vi "VISCOSITY_autoranging.vi"(1 "stabilization (ms)":u32=15000, 5 "TorqueOffset":dbl=-1.0, 6 "DataPoints":i32=10, 7 "GUID":string, 8 "Zero?":bool=TRUE, 9 "LogData?":bool=TRUE, 10 "rpm setpoint":i32=180) -> (0 "Torque% Offset":dbl, 2 "cP_mean":dbl format="%0.2f", 3 "TorqueArray":dbl[](array[numeric]), 4 "cP_Array":dbl[](array[numeric]))   [LabVIEW 2019]
uses:
  Brookfield_type-def.ctl
  <vilib>/Instr/_visa.llb/VISA Flush IO Buffer Mask.ctl
  <vilib>/Utility/error.llb/DialogType.ctl
  <vilib>/Analysis/baseanly.llb/Mean (DBL).vi
  <vilib>/Analysis/NI_AALBase.lvlib
panel:
  out "ReconnectAttempts":i32
  out "log_string":string
  out "error (enable read)":errorcluster
  out "TempArray":dbl[](array[numeric])
  out "error out":errorcluster
  out "Enum":T1
  out "temp":dbl
  out "torque%":dbl
  out "Control Circuitry Enabled":bool
  out "Motor On":bool
  out "Motor Stopped":bool
  out "Auto-zero Complete":bool
  out "Motor Circuit Error":bool
  out "Diagnostics Error":bool
  out "Invalid Command Received":bool
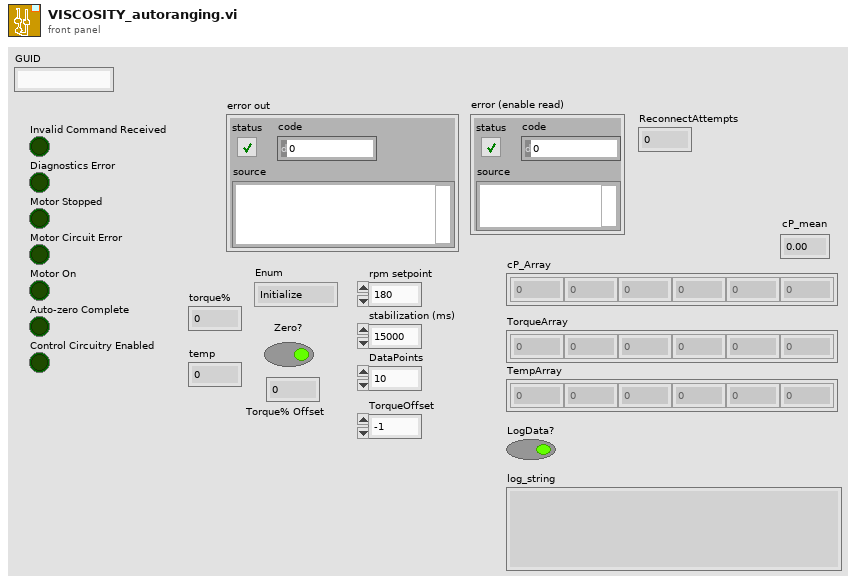
[diagram p1: front panel]
types:
  T1 = typedef "Brookfield_type-def.ctl" = enum16{"Initialize", "Enable", "Ready", "Zero", "Set Speed", "Read", "Stop Motor", "Error", "Disconnect"}
  T2 = enum16{"open", "replace", "create", "open or create", "replace or create", "replace or create with confirmation"}
  T3 = typedef "VISA Flush IO Buffer Mask.ctl" = u16
  T4 = typedef "DialogType.ctl" = u16
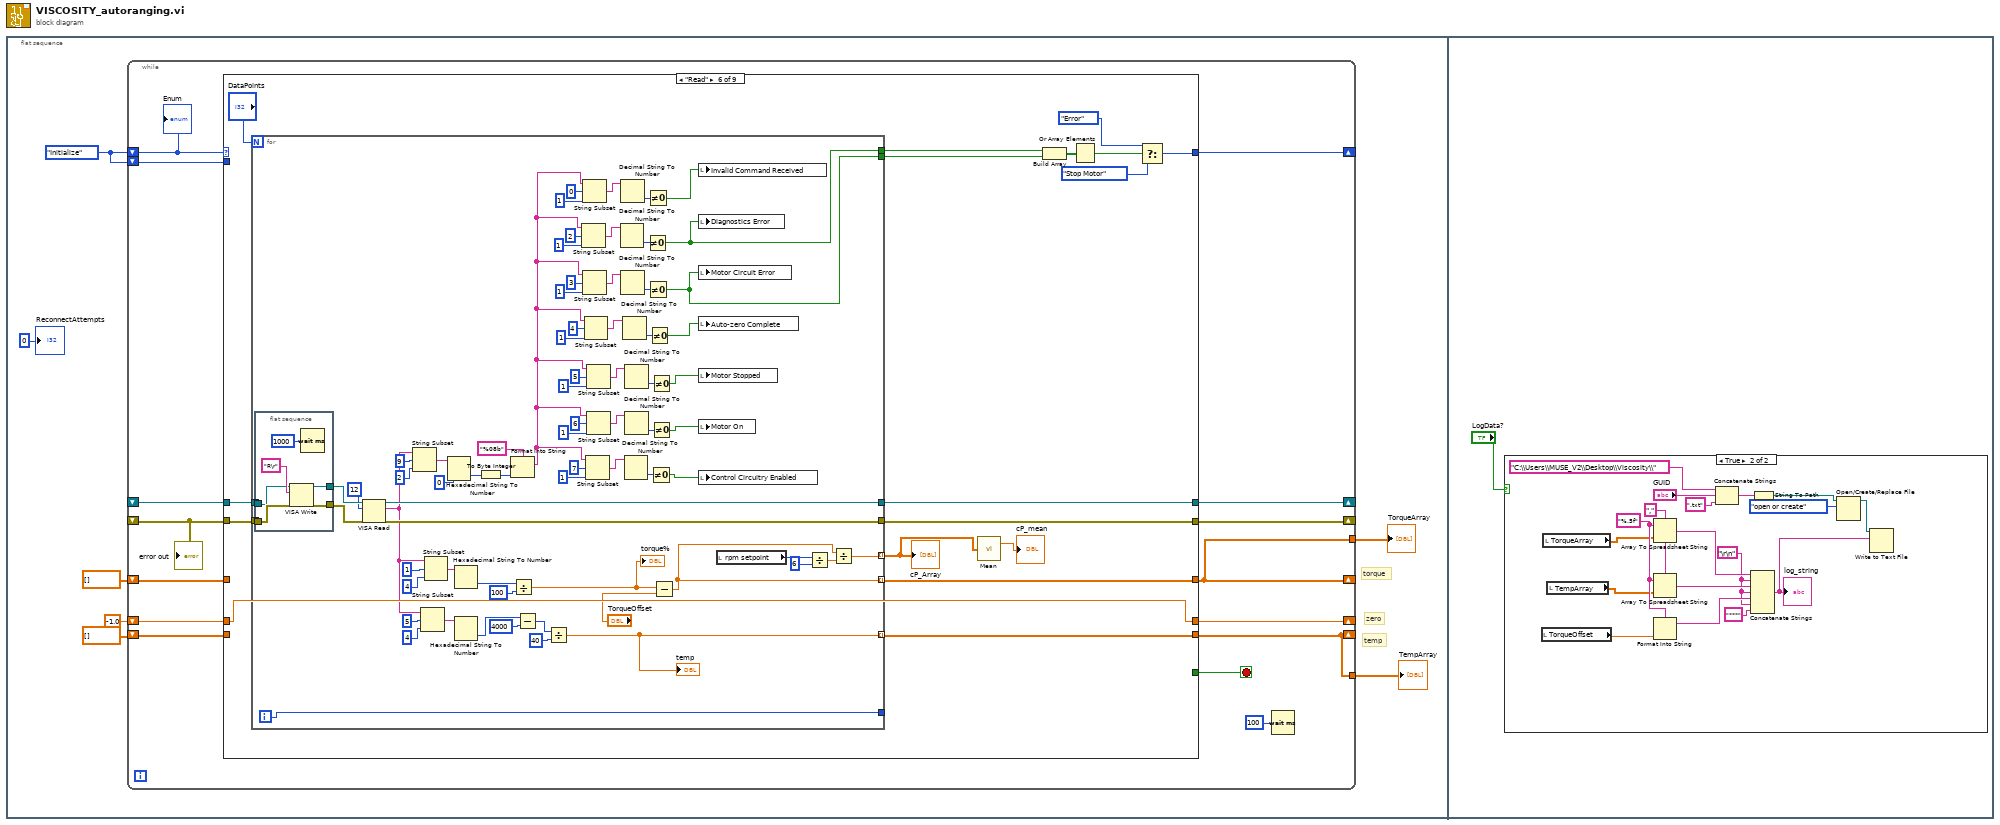
[diagram p0: block diagram]
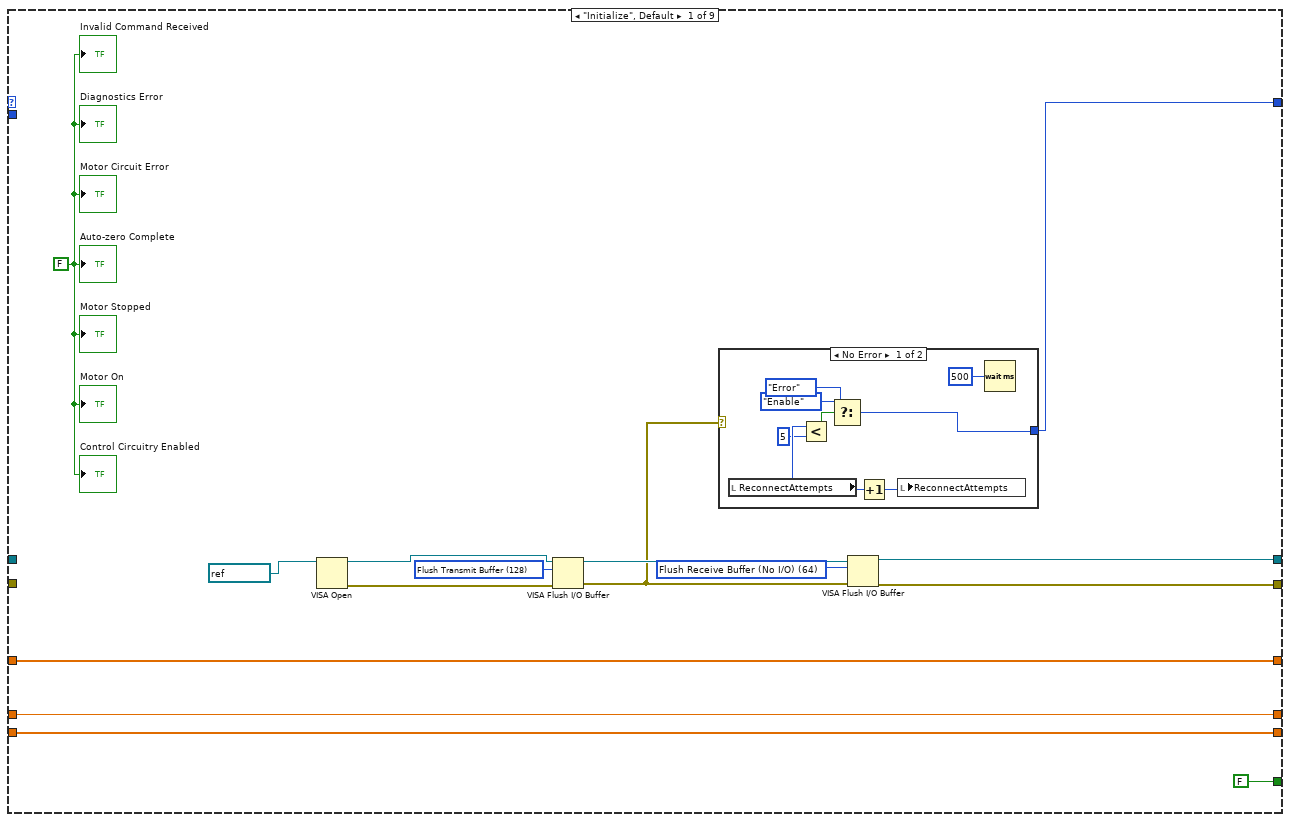
[diagram p2: hidden frame]
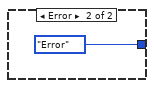
[diagram p3: hidden frame]
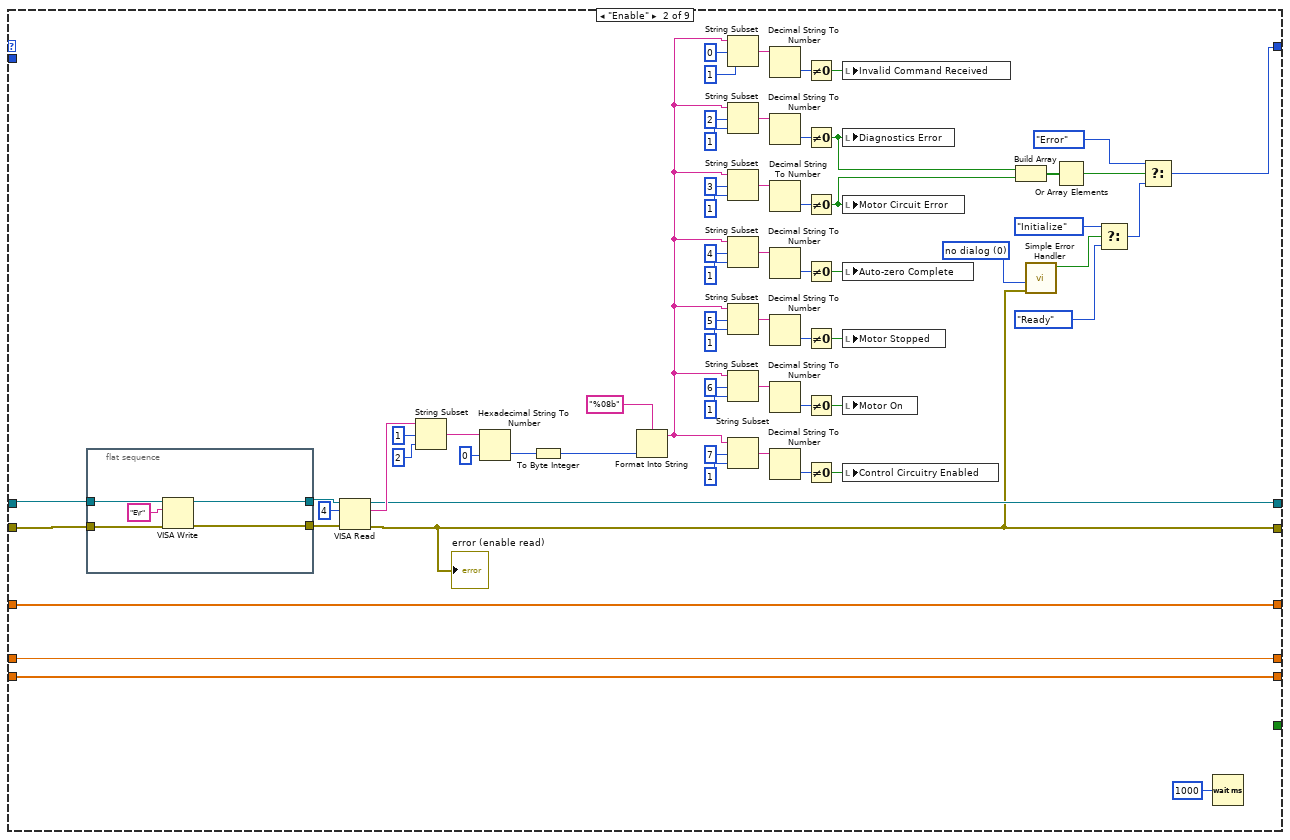
[diagram p4: hidden frame]
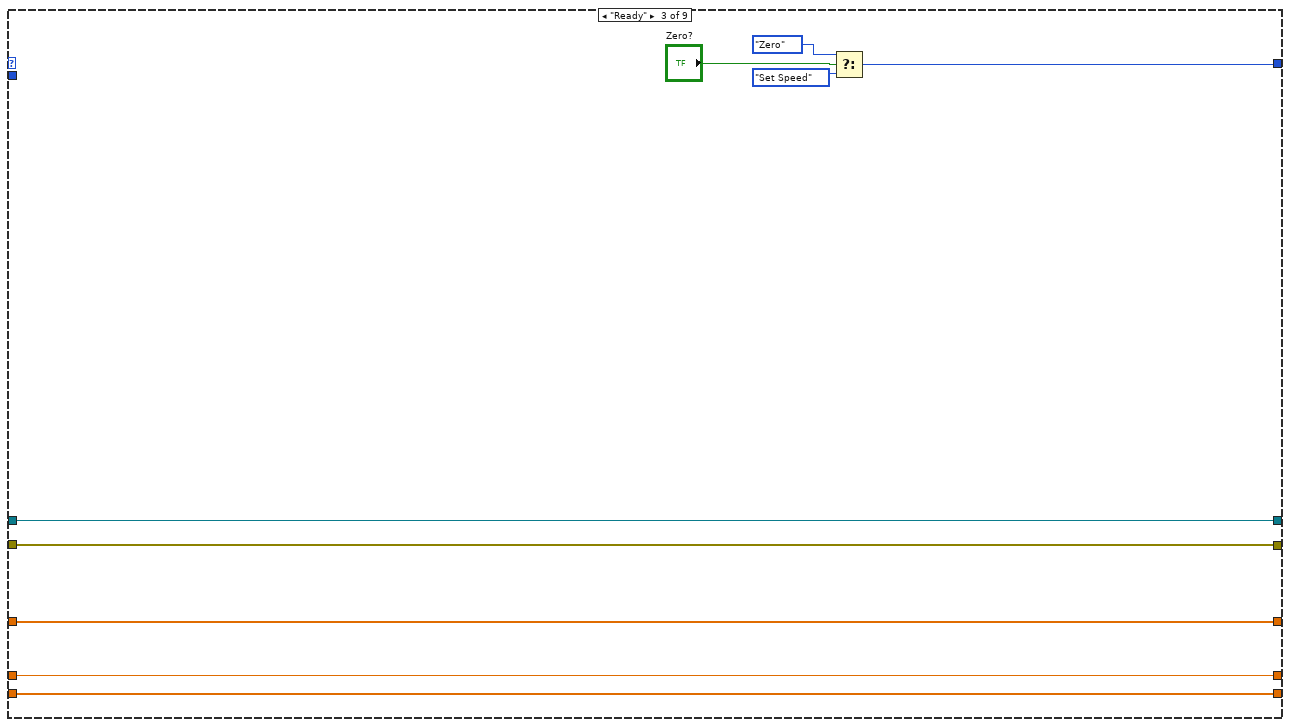
[diagram p5: hidden frame]
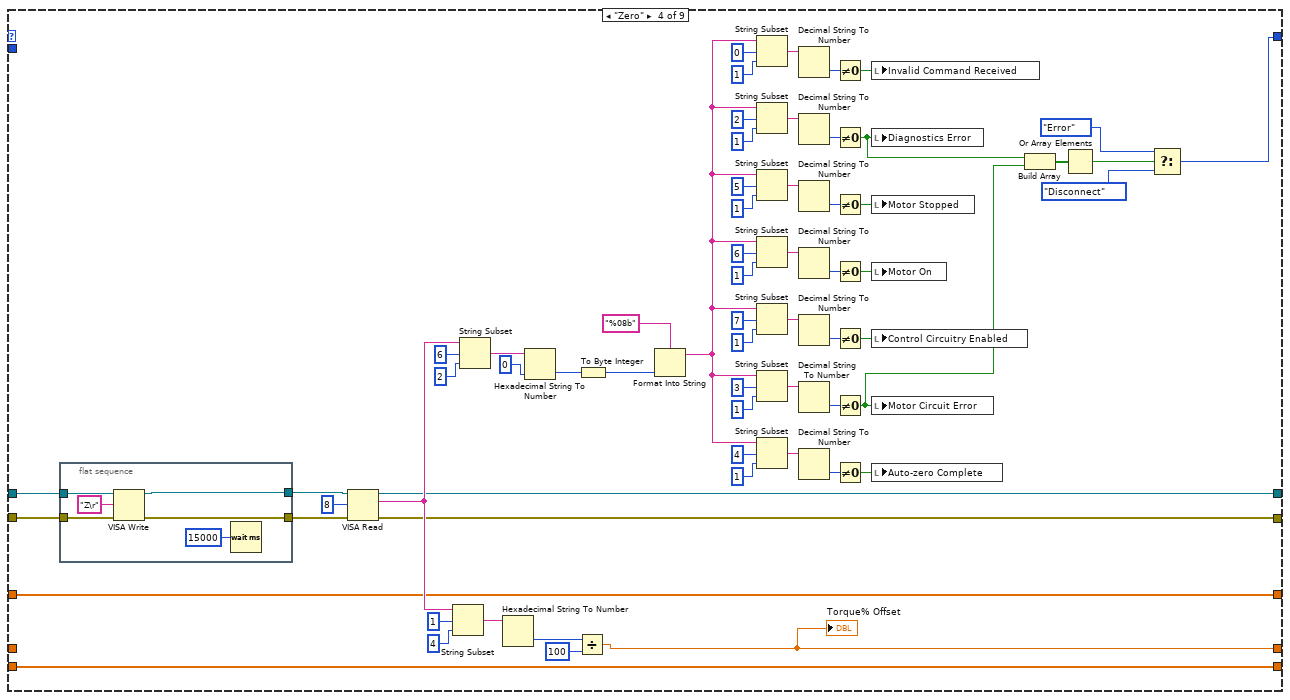
[diagram p6: hidden frame]
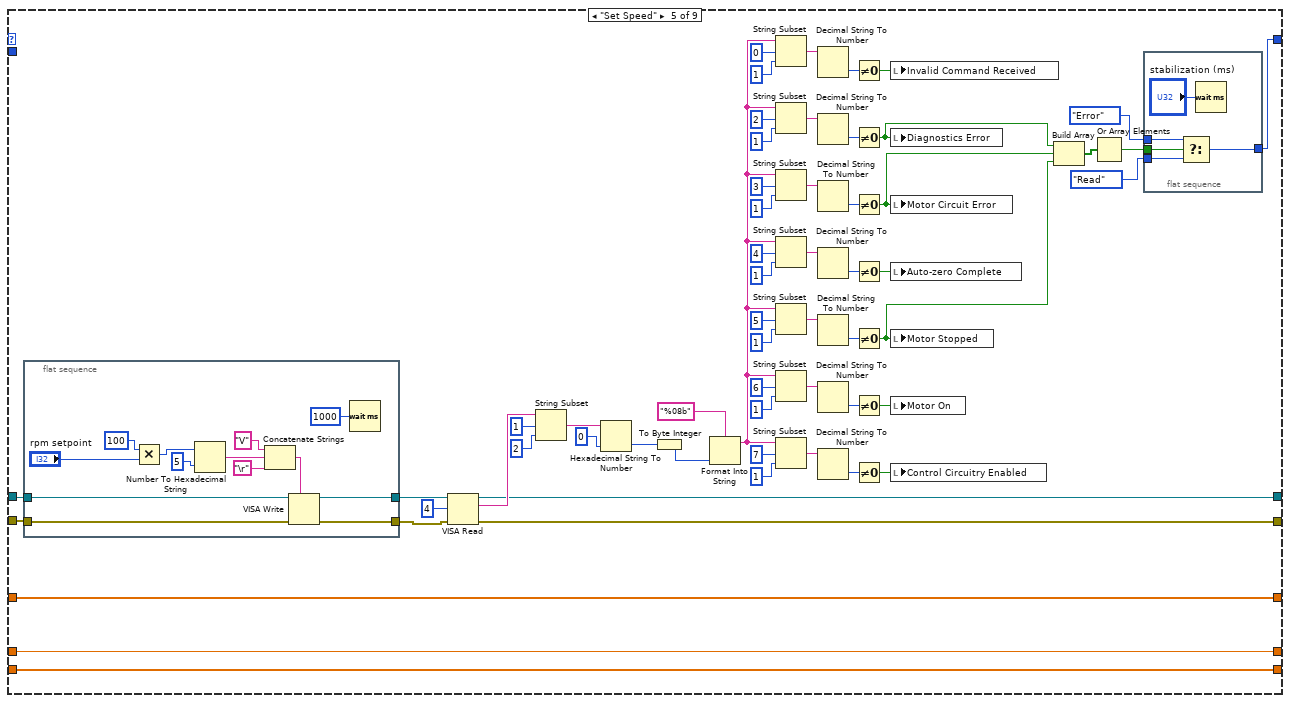
[diagram p7: hidden frame]
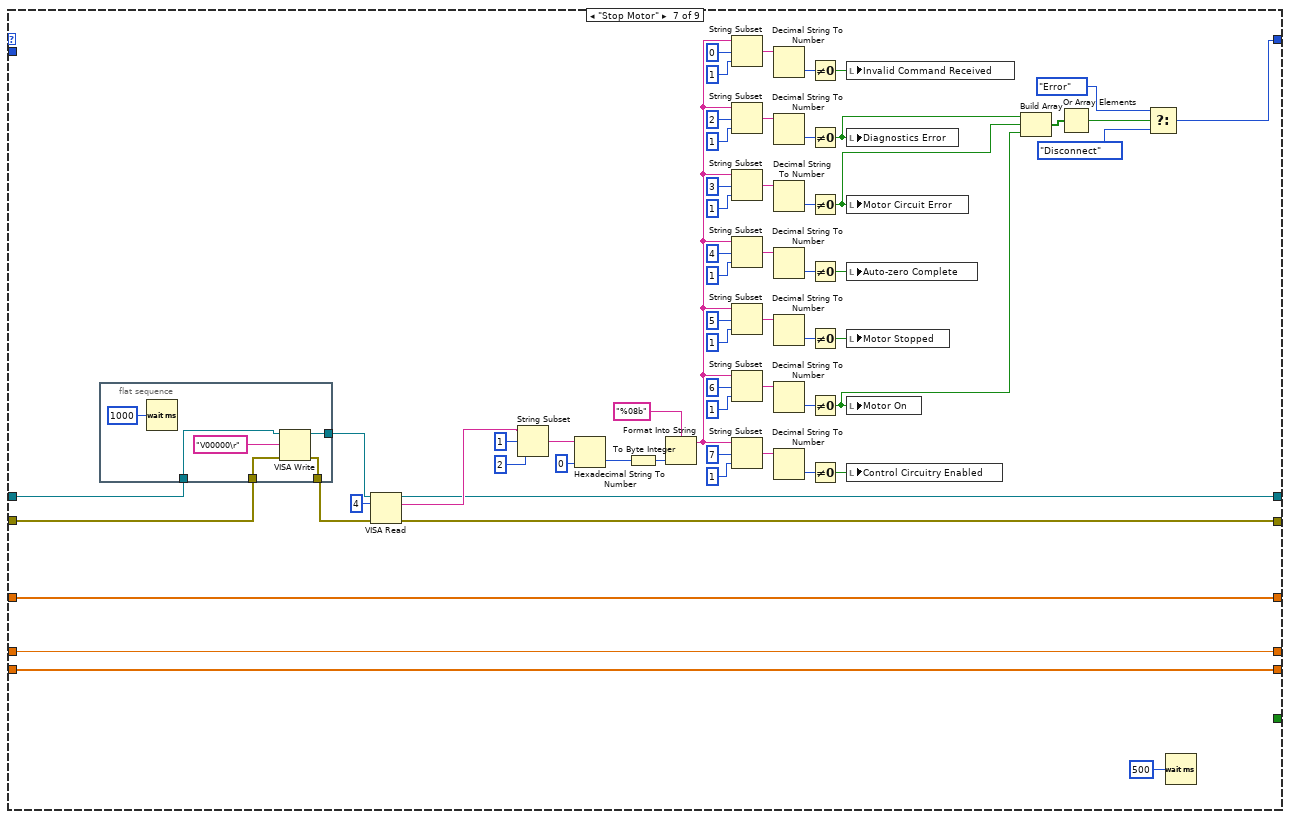
[diagram p8: hidden frame]
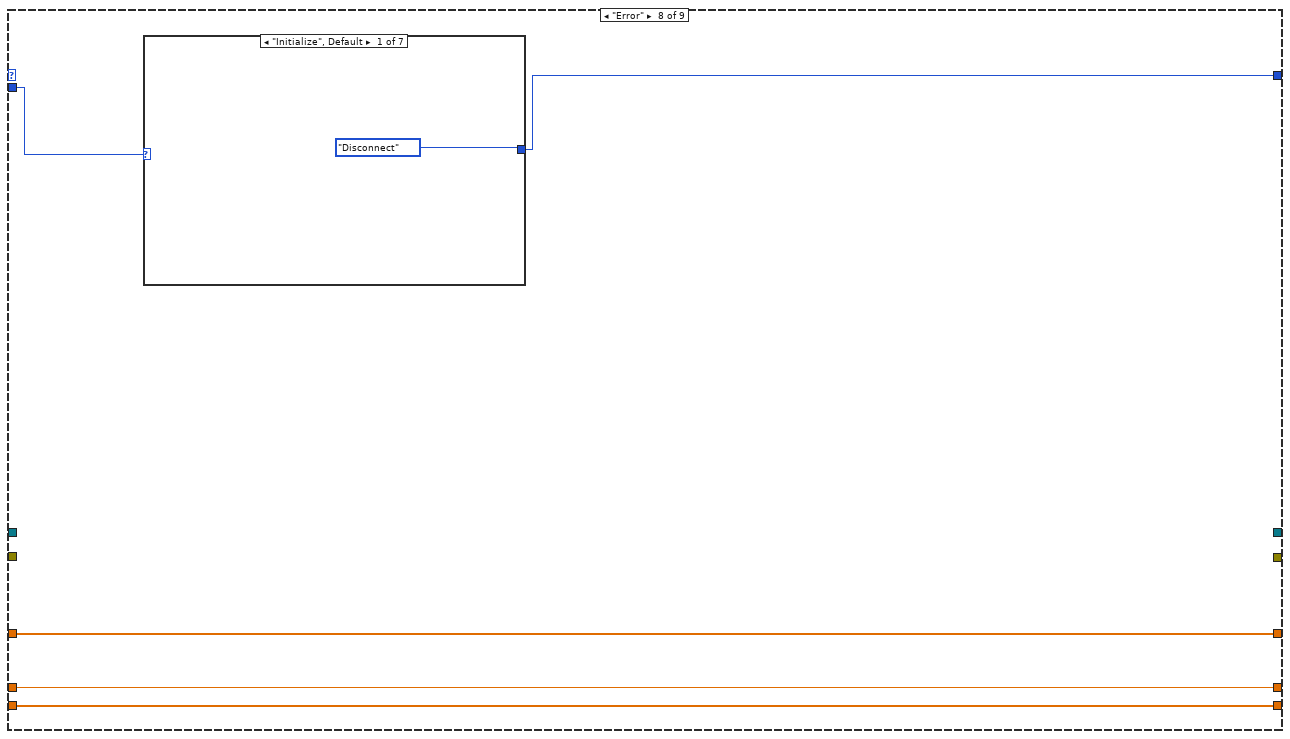
[diagram p9: hidden frame]
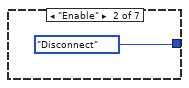
[diagram p10: hidden frame]
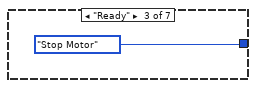
[diagram p11: hidden frame]
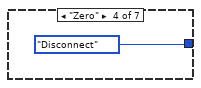
[diagram p12: hidden frame]
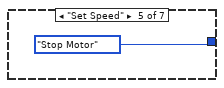
[diagram p13: hidden frame]
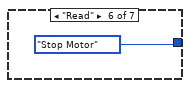
[diagram p14: hidden frame]
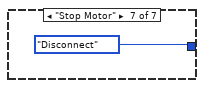
[diagram p15: hidden frame]
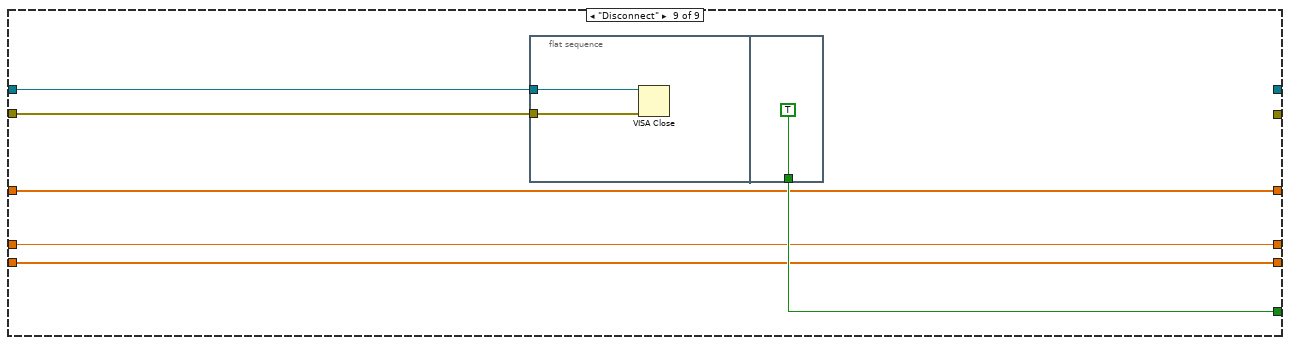
[diagram p16: hidden frame]
diagram:
  n1 = flat-sequence {
    frame #0 {
      w7 = Brookfield_type-def."Initialize"
      # "temp"
      # "zero"
      # "torque"
      n2 = while {
        shift-right: [w16] -> _
        shift-left: w7 -> [w22]
        shift-right: [w21] -> _
        shift-left: _ -> [w19]
        shift-right: [w20] -> _
        shift-left: _ -> [w18]
        shift-right: [w9] -> _
        shift-left: dbl[] [] -> [w14]
        shift-right: [w8] -> _
        shift-left: dbl[] [] -> [w11]
        shift-left: w7 -> [w15]
        shift-right: [w12] -> _
        shift-left: -1.0 -> [w13]
        tunnel: [w9] -> w3
        tunnel: [w8] -> w2
        stop <- w17 stop-if-true
        n3 = case shown="\"Read\"" w22 {
          tunnel: [w24 w65 w120 w135 w211 w288 w383 _ _] -> w21
          tunnel: [w23 w48 w121 w136 w212 w287 w384 _ _] -> w20
          tunnel: w19 -> [_ w110 w120 w138 w197 w276 w370 _ w450]
          tunnel: w18 -> [_ w109 w121 w137 w198 w277 w371 _ w449]
          tunnel: [FALSE _ _ _ _ _ _ _ w448] -> w17
          tunnel: [w34 w59 w117 w128 w206 w283 w378 w437 _] -> w16
          tunnel: [w33 w58 w124 w127 w201 w279 w374 w436 w447] -> w9
          tunnel: [w31 w56 w122 w126 w199 w280 w372 w434 w445] -> w8
          tunnel: [w32 w57 w123 w125 w200 w278 w373 w435 w446] -> w12
          tunnel: w15 -> [_ _ _ _ _ _ _ w433 _]
          tunnel: w14 -> [w33 w58 w124 w127 w201 _ w374 w436 w447]
          tunnel: w13 -> [w32 w57 w123 _ w200 w278 w373 w435 w446]
          tunnel: w11 -> [w31 w56 w122 w126 w199 _ w372 w434 w445]
          frame "Initialize", Default {
            w25 = T3 64 items=["Flush Receive Buffer"=16, "Write Transmit Buffer to Device"=32, "Flush Receive Buffer (No I/O)"=64, "Flush Transmit Buffer"=128] ("Mask")
            w28 = T3 128 items=["Flush Receive Buffer"=16, "Write Transmit Buffer to Device"=32, "Flush Receive Buffer (No I/O)"=64, "Flush Transmit Buffer"=128] ("Mask")
            w36 = FALSE
            n4 = VISA Open(VISA resource name=refnum<visa-resource-name> "COM5" ("Conductivity Port")) -> (VISA resource name=w29:refnum<visa-resource-name>, error out=w30:errorcluster)  [unwired: 4 in]
            n5 = VISA Flush I/O Buffer(VISA resource name=w29, mask (16)=w28, error in (no error)=w30) -> (VISA resource name out=w27:refnum<visa-resource-name>, error out=w26:errorcluster)
            n6 = case shown="No Error" w26 {
              tunnel: [w40 Brookfield_type-def."Error"] -> w34
              frame No Error {
                n7 = local read "ReconnectAttempts"() -> (w43:i32)
                n8 = Less?(x=w43, y=5) -> (x < y?=w41:bool)
                n9 = Select(t=Brookfield_type-def."Enable", s=w41, f=Brookfield_type-def."Error") -> (s? t:f=w40:T1)
                n10 = Increment(x=w43) -> (x+1=w44:i32)
                n11 = local write "ReconnectAttempts"(w44) -> ()
                n12 = Wait (ms)(milliseconds to wait=u32 500) -> ()  [unwired: 1 out]
              }
              frame Error {
              }
            }
            n13 = VISA Flush I/O Buffer(VISA resource name=w27, mask (16)=w25, error in (no error)=w26) -> (VISA resource name out=w24:refnum<visa-resource-name>, error out=w23:errorcluster)
            "Invalid Command Received" <- w36
            "Diagnostics Error" <- w36
            "Motor Circuit Error" <- w36
            "Auto-zero Complete" <- w36
            "Motor Stopped" <- w36
            "Motor On" <- w36
            "Control Circuitry Enabled" <- w36
          }
          frame "Enable" {
            w50 = T4 0 items=["no dialog", "OK message", "continue or stop message", "OK message + warnings", "continue/stop + warnings"] ("type of dialog (OK msg:1)")
            n14 = flat-sequence {
              tunnel: w110 -> [w114]
              tunnel: w109 -> [w113]
              tunnel: [w112] -> w49
              tunnel: [w111] -> w66
              frame #0 {
                n15 = VISA Write(VISA resource name=w114, write buffer="E\r", error in (no error)=w113) -> (VISA resource name out=w111:refnum<visa-resource-name>, error out=w112:errorcluster)  [unwired: 1 out]
              }
            }
            n16 = VISA Read(VISA resource name=w66, byte count=u32 4, error in (no error)=w49) -> (VISA resource name out=w65:refnum<visa-resource-name>, read buffer=w108:string, error out=w48:errorcluster)  [unwired: 1 out]
            "error (enable read)" <- w48
            n17 = String Subset(string=w108, offset (0)=1, length (rest)=2 ("length (rest)")) -> (substring=w102:string)
            n18 = Hexadecimal String To Number(string=w102, default (0uL)=u32 0 ("default (0 U32)")) -> (number=w98:u32)  [unwired: 1 in, 1 out]
            n19 = To Byte Integer(number=w98) -> (8bit integer=w99:i8)
            n20 = Format Into String(format string="%08b", w99) -> (resulting string=w85:string)  [unwired: 2 in, 1 out]
            n21 = String Subset(string=w85, offset (0)=0, length (rest)=1 ("length (rest)")) -> (substring=w101:string)
            n22 = String Subset(string=w85, offset (0)=2, length (rest)=1 ("length (rest)")) -> (substring=w96:string)
            n23 = String Subset(string=w85, offset (0)=3, length (rest)=1 ("length (rest)")) -> (substring=w95:string)
            n24 = String Subset(string=w85, offset (0)=4, length (rest)=1 ("length (rest)")) -> (substring=w92:string)
            n25 = String Subset(string=w85, offset (0)=5, length (rest)=1 ("length (rest)")) -> (substring=w91:string)
            n26 = String Subset(string=w85, offset (0)=6, length (rest)=1 ("length (rest)")) -> (substring=w88:string)
            n27 = String Subset(string=w85, offset (0)=7, length (rest)=1 ("length (rest)")) -> (substring=w87:string)
            n28 = Decimal String To Number(string=w101) -> (number=w100:i32)  [unwired: 2 in, 1 out]
            n29 = Decimal String To Number(string=w96) -> (number=w97:i32)  [unwired: 2 in, 1 out]
            n30 = Decimal String To Number(string=w95) -> (number=w94:i32)  [unwired: 2 in, 1 out]
            n31 = Decimal String To Number(string=w92) -> (number=w93:i32)  [unwired: 2 in, 1 out]
            n32 = Decimal String To Number(string=w91) -> (number=w90:i32)  [unwired: 2 in, 1 out]
            n33 = Decimal String To Number(string=w88) -> (number=w89:i32)  [unwired: 2 in, 1 out]
            n34 = Decimal String To Number(string=w87) -> (number=w86:i32)  [unwired: 2 in, 1 out]
            n35 = Not Equal To 0?(x=w100) -> (x != 0?=w103:bool)
            n36 = Not Equal To 0?(x=w97) -> (x != 0?=w64:bool)
            n37 = Not Equal To 0?(x=w94) -> (x != 0?=w63:bool)
            n38 = Not Equal To 0?(x=w93) -> (x != 0?=w104:bool)
            n39 = Not Equal To 0?(x=w90) -> (x != 0?=w105:bool)
            n40 = Not Equal To 0?(x=w89) -> (x != 0?=w106:bool)
            n41 = Not Equal To 0?(x=w86) -> (x != 0?=w107:bool)
            n42 = local write "Invalid Command Received"(w103) -> ()
            n43 = local write "Diagnostics Error"(w64) -> ()
            n44 = local write "Motor Circuit Error"(w63) -> ()
            n45 = local write "Auto-zero Complete"(w104) -> ()
            n46 = local write "Motor Stopped"(w105) -> ()
            n47 = local write "Motor On"(w106) -> ()
            n48 = local write "Control Circuitry Enabled"(w107) -> ()
            n49 = Build Array(w64, w63) -> (w62:bool[])
            n50 = call <vilib>:"Simple Error Handler.vi"("type of dialog (OK msg:1)"=w50, "error in (no error)"=w48) -> ("error?"=w52:bool)  [unwired: 3 in, 4 out]
            n51 = Or Array Elements(Boolean array=w62) -> (logical OR=w61:bool)
            n52 = Select(t=Brookfield_type-def."Initialize", s=w52, f=Brookfield_type-def."Ready") -> (s? t:f=w55:T1)
            n53 = Select(t=Brookfield_type-def."Error", s=w61, f=w55) -> (s? t:f=w59:T1)
            n54 = Wait (ms)(milliseconds to wait=u32 1000) -> ()  [unwired: 1 out]
          }
          frame "Ready" {
            n55 = Select(t=Brookfield_type-def."Zero", s="Zero?", f=Brookfield_type-def."Set Speed") -> (s? t:f=w117:T1)
          }
          frame "Zero" {
            n56 = flat-sequence {
              tunnel: [w194] -> w162
              tunnel: [w193] -> w161
              tunnel: w138 -> [w191]
              tunnel: w137 -> [w190]
              frame #0 {
                n57 = VISA Write(VISA resource name=w191, write buffer="Z\r", error in (no error)=w190) -> (VISA resource name out=w193:refnum<visa-resource-name>, error out=w194:errorcluster)  [unwired: 1 out]
                n58 = Wait (ms)(milliseconds to wait=u32 15000) -> ()  [unwired: 1 out]
              }
            }
            n59 = VISA Read(VISA resource name=w161, byte count=u32 8, error in (no error)=w162) -> (VISA resource name out=w135:refnum<visa-resource-name>, read buffer=w183:string, error out=w136:errorcluster)  [unwired: 1 out]
            n60 = String Subset(string=w183, offset (0)=1, length (rest)=4 ("length (rest)")) -> (substring=w163:string)
            n61 = String Subset(string=w183, offset (0)=6, length (rest)=2 ("length (rest)")) -> (substring=w165:string)
            n62 = Hexadecimal String To Number(string=w163) -> (number=w164:u32)  [unwired: 2 in, 1 out]
            n63 = Hexadecimal String To Number(string=w165, default (0uL)=u32 0 ("default (0 U32)")) -> (number=w169:u32)  [unwired: 1 in, 1 out]
            n64 = Divide(x=w164, y=u32 100) -> (x/y=w125:dbl)
            "Torque% Offset" <- w125
            n65 = To Byte Integer(number=w169) -> (8bit integer=w168:i8)
            n66 = Format Into String(format string="%08b", w168) -> (resulting string=w182:string)  [unwired: 2 in, 1 out]
            n67 = String Subset(string=w182, offset (0)=0, length (rest)=1 ("length (rest)")) -> (substring=w166:string)
            n68 = String Subset(string=w182, offset (0)=2, length (rest)=1 ("length (rest)")) -> (substring=w171:string)
            n69 = String Subset(string=w182, offset (0)=5, length (rest)=1 ("length (rest)")) -> (substring=w176:string)
            n70 = String Subset(string=w182, offset (0)=6, length (rest)=1 ("length (rest)")) -> (substring=w179:string)
            n71 = String Subset(string=w182, offset (0)=7, length (rest)=1 ("length (rest)")) -> (substring=w180:string)
            n72 = String Subset(string=w182, offset (0)=3, length (rest)=1 ("length (rest)")) -> (substring=w172:string)
            n73 = String Subset(string=w182, offset (0)=4, length (rest)=1 ("length (rest)")) -> (substring=w175:string)
            n74 = Decimal String To Number(string=w166) -> (number=w167:i32)  [unwired: 2 in, 1 out]
            n75 = Decimal String To Number(string=w171) -> (number=w170:i32)  [unwired: 2 in, 1 out]
            n76 = Decimal String To Number(string=w176) -> (number=w177:i32)  [unwired: 2 in, 1 out]
            n77 = Decimal String To Number(string=w179) -> (number=w178:i32)  [unwired: 2 in, 1 out]
            n78 = Decimal String To Number(string=w180) -> (number=w181:i32)  [unwired: 2 in, 1 out]
            n79 = Decimal String To Number(string=w172) -> (number=w173:i32)  [unwired: 2 in, 1 out]
            n80 = Decimal String To Number(string=w175) -> (number=w174:i32)  [unwired: 2 in, 1 out]
            n81 = Not Equal To 0?(x=w167) -> (x != 0?=w188:bool)
            n82 = Not Equal To 0?(x=w170) -> (x != 0?=w130:bool)
            n83 = Not Equal To 0?(x=w177) -> (x != 0?=w186:bool)
            n84 = Not Equal To 0?(x=w178) -> (x != 0?=w185:bool)
            n85 = Not Equal To 0?(x=w181) -> (x != 0?=w184:bool)
            n86 = Not Equal To 0?(x=w173) -> (x != 0?=w129:bool)
            n87 = Not Equal To 0?(x=w174) -> (x != 0?=w187:bool)
            n88 = local write "Invalid Command Received"(w188) -> ()
            n89 = local write "Diagnostics Error"(w130) -> ()
            n90 = local write "Motor Stopped"(w186) -> ()
            n91 = local write "Motor On"(w185) -> ()
            n92 = local write "Control Circuitry Enabled"(w184) -> ()
            n93 = local write "Motor Circuit Error"(w129) -> ()
            n94 = local write "Auto-zero Complete"(w187) -> ()
            n95 = Build Array(w130, w129) -> (w134:bool[])
            n96 = Or Array Elements(Boolean array=w134) -> (logical OR=w133:bool)
            n97 = Select(t=Brookfield_type-def."Error", s=w133, f=Brookfield_type-def."Disconnect") -> (s? t:f=w128:T1)
          }
          frame "Set Speed" {
            n98 = flat-sequence {
              tunnel: w198 -> [w262]
              tunnel: w197 -> [w261]
              tunnel: [w260] -> w196
              tunnel: [w259] -> w195
              frame #0 {
                n99 = Multiply(x=100, y="rpm setpoint") -> (x*y=w269:i32)
                n100 = Number To Hexadecimal String(1:i16 5 ("width (-)"), 2:w269) -> (0:w268:string)
                n101 = Concatenate Strings("V" ("string"), w268, "\r") -> (w267:string)
                n102 = VISA Write(VISA resource name=w261, write buffer=w267, error in (no error)=w262) -> (VISA resource name out=w259:refnum<visa-resource-name>, error out=w260:errorcluster)  [unwired: 1 out]
                n103 = Wait (ms)(milliseconds to wait=u32 1000) -> ()  [unwired: 1 out]
              }
            }
            n104 = VISA Read(VISA resource name=w195, byte count=u32 4, error in (no error)=w196) -> (VISA resource name out=w211:refnum<visa-resource-name>, read buffer=w253:string, error out=w212:errorcluster)  [unwired: 1 out]
            n105 = String Subset(string=w253, offset (0)=1, length (rest)=2 ("length (rest)")) -> (substring=w249:string)
            n106 = Hexadecimal String To Number(string=w249, default (0uL)=u32 0 ("default (0 U32)")) -> (number=w245:u32)  [unwired: 1 in, 1 out]
            n107 = To Byte Integer(number=w245) -> (8bit integer=w246:i8)
            n108 = Format Into String(format string="%08b", w246) -> (resulting string=w232:string)  [unwired: 2 in, 1 out]
            n109 = String Subset(string=w232, offset (0)=0, length (rest)=1 ("length (rest)")) -> (substring=w248:string)
            n110 = String Subset(string=w232, offset (0)=2, length (rest)=1 ("length (rest)")) -> (substring=w243:string)
            n111 = String Subset(string=w232, offset (0)=3, length (rest)=1 ("length (rest)")) -> (substring=w242:string)
            n112 = String Subset(string=w232, offset (0)=4, length (rest)=1 ("length (rest)")) -> (substring=w239:string)
            n113 = String Subset(string=w232, offset (0)=5, length (rest)=1 ("length (rest)")) -> (substring=w238:string)
            n114 = String Subset(string=w232, offset (0)=6, length (rest)=1 ("length (rest)")) -> (substring=w235:string)
            n115 = String Subset(string=w232, offset (0)=7, length (rest)=1 ("length (rest)")) -> (substring=w234:string)
            n116 = Decimal String To Number(string=w248) -> (number=w247:i32)  [unwired: 2 in, 1 out]
            n117 = Decimal String To Number(string=w243) -> (number=w244:i32)  [unwired: 2 in, 1 out]
            n118 = Decimal String To Number(string=w242) -> (number=w241:i32)  [unwired: 2 in, 1 out]
            n119 = Decimal String To Number(string=w239) -> (number=w240:i32)  [unwired: 2 in, 1 out]
            n120 = Decimal String To Number(string=w238) -> (number=w237:i32)  [unwired: 2 in, 1 out]
            n121 = Decimal String To Number(string=w235) -> (number=w236:i32)  [unwired: 2 in, 1 out]
            n122 = Decimal String To Number(string=w234) -> (number=w233:i32)  [unwired: 2 in, 1 out]
            n123 = Not Equal To 0?(x=w247) -> (x != 0?=w250:bool)
            n124 = Not Equal To 0?(x=w244) -> (x != 0?=w204:bool)
            n125 = Not Equal To 0?(x=w241) -> (x != 0?=w205:bool)
            n126 = Not Equal To 0?(x=w240) -> (x != 0?=w251:bool)
            n127 = Not Equal To 0?(x=w237) -> (x != 0?=w202:bool)
            n128 = Not Equal To 0?(x=w236) -> (x != 0?=w203:bool)
            n129 = Not Equal To 0?(x=w233) -> (x != 0?=w252:bool)
            n130 = local write "Invalid Command Received"(w250) -> ()
            n131 = local write "Diagnostics Error"(w204) -> ()
            n132 = local write "Motor Circuit Error"(w205) -> ()
            n133 = local write "Auto-zero Complete"(w251) -> ()
            n134 = local write "Motor Stopped"(w202) -> ()
            n135 = local write "Motor On"(w203) -> ()
            n136 = local write "Control Circuitry Enabled"(w252) -> ()
            n137 = Build Array(w204, w205, w202) -> (w210:bool[])
            n138 = Or Array Elements(Boolean array=w210) -> (logical OR=w209:bool)
            n139 = flat-sequence {
              tunnel: w209 -> [w258]
              tunnel: Brookfield_type-def."Read" -> [w257]
              tunnel: Brookfield_type-def."Error" -> [w256]
              tunnel: [w255] -> w206
              frame #0 {
                n140 = Select(t=w256, s=w258, f=w257) -> (s? t:f=w255:T1)
                n141 = Wait (ms)(milliseconds to wait="stabilization (ms)") -> ()  [unwired: 1 out]
              }
            }
          }
          frame "Read" {
            n142 = for {
              N: "DataPoints" -> [_]
              tunnel: [w360] -> w288
              tunnel: [w359] -> w287
              tunnel: [w358] -> w282
              tunnel: [w357] -> w281
              tunnel: [w356] -> w280 mode=indexing
              tunnel: [w291] -> w279 mode=indexing
              tunnel: w277 -> [w355]
              tunnel: w276 -> [w354]
              tunnel: [w296] -> _
              tunnel: [w290] -> w273 mode=indexing
              i -> [w296]
              n143 = flat-sequence {
                tunnel: w355 -> [w365]
                tunnel: w354 -> [w363]
                tunnel: [w362] -> w353
                tunnel: [w361] -> w352
                frame #0 {
                  n144 = VISA Write(VISA resource name=w363, write buffer="R\r", error in (no error)=w365) -> (VISA resource name out=w361:refnum<visa-resource-name>, error out=w362:errorcluster)  [unwired: 1 out]
                  n145 = Wait (ms)(milliseconds to wait=u32 1000) -> ()  [unwired: 1 out]
                }
              }
              n146 = VISA Read(VISA resource name=w352, byte count=u32 12, error in (no error)=w353) -> (VISA resource name out=w360:refnum<visa-resource-name>, read buffer=w336:string, error out=w359:errorcluster)  [unwired: 1 out]
              n147 = String Subset(string=w336, offset (0)=9, length (rest)=2 ("length (rest)")) -> (substring=w335:string)
              n148 = String Subset(string=w336, offset (0)=5, length (rest)=4 ("length (rest)")) -> (substring=w342:string)
              n149 = String Subset(string=w336, offset (0)=1, length (rest)=4 ("length (rest)")) -> (substring=w348:string)
              n150 = Hexadecimal String To Number(string=w335, default (0uL)=u32 0 ("default (0 U32)")) -> (number=w327:u32)  [unwired: 1 in, 1 out]
              n151 = Hexadecimal String To Number(string=w348) -> (number=w347:u32)  [unwired: 2 in, 1 out]
              n152 = Hexadecimal String To Number(string=w342) -> (number=w341:u32)  [unwired: 2 in, 1 out]
              n153 = To Byte Integer(number=w327) -> (8bit integer=w328:i8)
              n154 = Format Into String(format string="%08b", w328) -> (resulting string=w302:string)  [unwired: 2 in, 1 out]
              n155 = Divide(x=w347, y=u32 100) -> (x/y=w295:dbl)
              "torque%" <- w295
              n156 = Subtract(x=w341, y=u32 4000) -> (x-y=w339:u32)
              n157 = Divide(x=w339, y=u32 40) -> (x/y=w356:dbl)
              "temp" <- w356
              n158 = String Subset(string=w302, offset (0)=2, length (rest)=1 ("length (rest)")) -> (substring=w325:string)
              n159 = String Subset(string=w302, offset (0)=0, length (rest)=1 ("length (rest)")) -> (substring=w331:string)
              n160 = String Subset(string=w302, offset (0)=3, length (rest)=1 ("length (rest)")) -> (substring=w320:string)
              n161 = String Subset(string=w302, offset (0)=4, length (rest)=1 ("length (rest)")) -> (substring=w317:string)
              n162 = String Subset(string=w302, offset (0)=7, length (rest)=1 ("length (rest)")) -> (substring=w304:string)
              n163 = String Subset(string=w302, offset (0)=5, length (rest)=1 ("length (rest)")) -> (substring=w312:string)
              n164 = String Subset(string=w302, offset (0)=6, length (rest)=1 ("length (rest)")) -> (substring=w309:string)
              n165 = Decimal String To Number(string=w325) -> (number=w326:i32)  [unwired: 2 in, 1 out]
              n166 = Decimal String To Number(string=w331) -> (number=w330:i32)  [unwired: 2 in, 1 out]
              n167 = Decimal String To Number(string=w320) -> (number=w319:i32)  [unwired: 2 in, 1 out]
              n168 = Decimal String To Number(string=w317) -> (number=w318:i32)  [unwired: 2 in, 1 out]
              n169 = Decimal String To Number(string=w304) -> (number=w303:i32)  [unwired: 2 in, 1 out]
              n170 = Decimal String To Number(string=w312) -> (number=w311:i32)  [unwired: 2 in, 1 out]
              n171 = Decimal String To Number(string=w309) -> (number=w310:i32)  [unwired: 2 in, 1 out]
              n172 = Not Equal To 0?(x=w326) -> (x != 0?=w358:bool)
              n173 = Not Equal To 0?(x=w330) -> (x != 0?=w297:bool)
              n174 = Not Equal To 0?(x=w319) -> (x != 0?=w357:bool)
              n175 = Not Equal To 0?(x=w318) -> (x != 0?=w298:bool)
              n176 = Not Equal To 0?(x=w303) -> (x != 0?=w301:bool)
              n177 = Not Equal To 0?(x=w311) -> (x != 0?=w299:bool)
              n178 = Not Equal To 0?(x=w310) -> (x != 0?=w300:bool)
              n179 = Subtract(x=w295, y="TorqueOffset") -> (x-y=w291:dbl)
              n180 = local write "Invalid Command Received"(w297) -> ()
              n181 = local write "Diagnostics Error"(w358) -> ()
              n182 = local write "Motor Circuit Error"(w357) -> ()
              n183 = local write "Auto-zero Complete"(w298) -> ()
              n184 = local write "Motor Stopped"(w299) -> ()
              n185 = local write "Motor On"(w300) -> ()
              n186 = local write "Control Circuitry Enabled"(w301) -> ()
              n187 = local read "rpm setpoint"() -> (w294:i32)
              n188 = Divide(x=w294, y=6) -> (x/y=w292:dbl)
              n189 = Divide(x=w291, y=w292) -> (x/y=w290:dbl)
            }
            "cP_Array" <- w273
            n190 = call-poly <vilib>:"Mean.vi"("X"=w273) -> ("mean"=→"cP_mean":dbl)  [unwired: 1 out]
            n191 = Build Array(w282, w281) -> (w284:bool[])
            n192 = Or Array Elements(Boolean array=w284) -> (logical OR=w286:bool)
            n193 = Select(t=Brookfield_type-def."Error", s=w286, f=Brookfield_type-def."Stop Motor") -> (s? t:f=w283:T1)
          }
          frame "Stop Motor" {
            n194 = flat-sequence {
              tunnel: w371 -> [w431]
              tunnel: w370 -> [w429]
              tunnel: [w428] -> w369
              tunnel: [w427] -> w368
              frame #0 {
                n195 = Wait (ms)(milliseconds to wait=u32 1000) -> ()  [unwired: 1 out]
                n196 = VISA Write(VISA resource name=w429, write buffer="V00000\r", error in (no error)=w431) -> (VISA resource name out=w427:refnum<visa-resource-name>, error out=w428:errorcluster)  [unwired: 1 out]
              }
            }
            n197 = VISA Read(VISA resource name=w368, byte count=u32 4, error in (no error)=w369) -> (VISA resource name out=w383:refnum<visa-resource-name>, read buffer=w404:string, error out=w384:errorcluster)  [unwired: 1 out]
            n198 = String Subset(string=w404, offset (0)=1, length (rest)=2 ("length (rest)")) -> (substring=w409:string)
            n199 = Hexadecimal String To Number(string=w409, default (0uL)=u32 0 ("default (0 U32)")) -> (number=w413:u32)  [unwired: 1 in, 1 out]
            n200 = To Byte Integer(number=w413) -> (8bit integer=w412:i8)
            n201 = Format Into String(format string="%08b", w412) -> (resulting string=w426:string)  [unwired: 2 in, 1 out]
            n202 = String Subset(string=w426, offset (0)=0, length (rest)=1 ("length (rest)")) -> (substring=w410:string)
            n203 = String Subset(string=w426, offset (0)=2, length (rest)=1 ("length (rest)")) -> (substring=w415:string)
            n204 = String Subset(string=w426, offset (0)=3, length (rest)=1 ("length (rest)")) -> (substring=w416:string)
            n205 = String Subset(string=w426, offset (0)=4, length (rest)=1 ("length (rest)")) -> (substring=w419:string)
            n206 = String Subset(string=w426, offset (0)=5, length (rest)=1 ("length (rest)")) -> (substring=w420:string)
            n207 = String Subset(string=w426, offset (0)=6, length (rest)=1 ("length (rest)")) -> (substring=w423:string)
            n208 = String Subset(string=w426, offset (0)=7, length (rest)=1 ("length (rest)")) -> (substring=w424:string)
            n209 = Decimal String To Number(string=w410) -> (number=w411:i32)  [unwired: 2 in, 1 out]
            n210 = Decimal String To Number(string=w415) -> (number=w414:i32)  [unwired: 2 in, 1 out]
            n211 = Decimal String To Number(string=w416) -> (number=w417:i32)  [unwired: 2 in, 1 out]
            n212 = Decimal String To Number(string=w419) -> (number=w418:i32)  [unwired: 2 in, 1 out]
            n213 = Decimal String To Number(string=w420) -> (number=w421:i32)  [unwired: 2 in, 1 out]
            n214 = Decimal String To Number(string=w423) -> (number=w422:i32)  [unwired: 2 in, 1 out]
            n215 = Decimal String To Number(string=w424) -> (number=w425:i32)  [unwired: 2 in, 1 out]
            n216 = Not Equal To 0?(x=w411) -> (x != 0?=w408:bool)
            n217 = Not Equal To 0?(x=w414) -> (x != 0?=w377:bool)
            n218 = Not Equal To 0?(x=w417) -> (x != 0?=w376:bool)
            n219 = Not Equal To 0?(x=w418) -> (x != 0?=w407:bool)
            n220 = Not Equal To 0?(x=w421) -> (x != 0?=w406:bool)
            n221 = Not Equal To 0?(x=w422) -> (x != 0?=w375:bool)
            n222 = Not Equal To 0?(x=w425) -> (x != 0?=w405:bool)
            n223 = local write "Invalid Command Received"(w408) -> ()
            n224 = local write "Diagnostics Error"(w377) -> ()
            n225 = local write "Motor Circuit Error"(w376) -> ()
            n226 = local write "Auto-zero Complete"(w407) -> ()
            n227 = local write "Motor Stopped"(w406) -> ()
            n228 = local write "Motor On"(w375) -> ()
            n229 = local write "Control Circuitry Enabled"(w405) -> ()
            n230 = Build Array(w377, w376, w375) -> (w382:bool[])
            n231 = Or Array Elements(Boolean array=w382) -> (logical OR=w381:bool)
            n232 = Select(t=Brookfield_type-def."Error", s=w381, f=Brookfield_type-def."Disconnect") -> (s? t:f=w378:T1)
            n233 = Wait (ms)(milliseconds to wait=u32 500) -> ()  [unwired: 1 out]
          }
          frame "Error" {
            n234 = case shown="\"Initialize\", Default" w433 {
              tunnel: [Brookfield_type-def."Disconnect" Brookfield_type-def."Disconnect" Brookfield_type-def."Stop Motor" Brookfield_type-def."Disconnect" Brookfield_type-def."Stop Motor" Brookfield_type-def."Stop Motor" Brookfield_type-def."Disconnect"] -> w437
              frame "Initialize", Default {
              }
              frame "Enable" {
              }
              frame "Ready" {
              }
              frame "Zero" {
              }
              frame "Set Speed" {
              }
              frame "Read" {
              }
              frame "Stop Motor" {
              }
            }
          }
          frame "Disconnect" {
            n235 = flat-sequence {
              tunnel: w450 -> [w452]
              tunnel: w449 -> [w451]
              tunnel: [TRUE] -> w448
              frame #0 {
                n236 = VISA Close(VISA resource name=w452, error in (no error)=w451) -> ()  [unwired: 1 out]
              }
              frame #1 {
              }
            }
          }
        }
        n237 = Wait (ms)(milliseconds to wait=u32 100) -> ()  [unwired: 1 out]
        "Enum" <- w22
        "error out" <- w18
      }
      "TorqueArray" <- w3
      "TempArray" <- w2
      "ReconnectAttempts" <- 0
    }
    frame #1 {
      n238 = case shown="True" "LogData?" {
        frame False {
        }
        frame True {
          w459 = "\r\n"
          w460 = "," ("delimiter (Tab)")
          w461 = "%.5f" ("format (%.3f)")
          n239 = local read "TorqueOffset"() -> (w457:dbl)
          n240 = local read "TorqueArray"() -> (w455:dbl[])
          n241 = local read "TempArray"() -> (w456:dbl[])
          n242 = Array To Spreadsheet String(delimiter (Tab)=w460, array=w455, 3:w461) -> (spreadsheet string=w465:string)
          n243 = Array To Spreadsheet String(delimiter (Tab)=w460, array=w456, 3:w461) -> (spreadsheet string=w464:string)
          n244 = Format Into String(format string=w461, w457) -> (resulting string=w463:string)  [unwired: 2 in, 1 out]
          n245 = Concatenate Strings("C:\\Users\\MUSE_V2\\Desktop\\Viscosity\\", "GUID", ".txt" ("string")) -> (w470:string)
          n246 = Concatenate Strings(w465, w459, w464, w459, w463, w459, "***" ("string")) -> (w462:string)
          "log_string" <- w462
          n247 = String To Path(string=w470) -> (path=w468:path)
          n248 = Open/Create/Replace File(file path (use dialog)=w468, operation (0:open)=T2."open or create") -> (refnum out=w469:refnum<file>)  [unwired: 4 in, 2 out]
          n249 = Write to Text File(file (use dialog)=w469, text=w462) -> ()  [unwired: 2 in, 3 out]
        }
      }
    }
  }
